vi "RelayBoard_ReadDi.vi"(9 "VISA资源名称":refnum<visa-resource-name>, 10 "比较值":bool, 11 "索引":i32) -> (2 "结果":bool, 3 "数组":bool[](array[boolean]))   [LabVIEW 2013]
panel:
  out "读取缓冲区":string
  # "深圳市德蓝新能源有限公司"
  # "X1"
  # "X2"
  # "X3"
  # "X4"
  # "X5"
  # "X6"
  # "X7"
  # "X8"
  # "X9"
  # "X10"
  # "X11"
  # "X12"
  # "X13"
  # "X14"
  # "X15"
  # "X16"
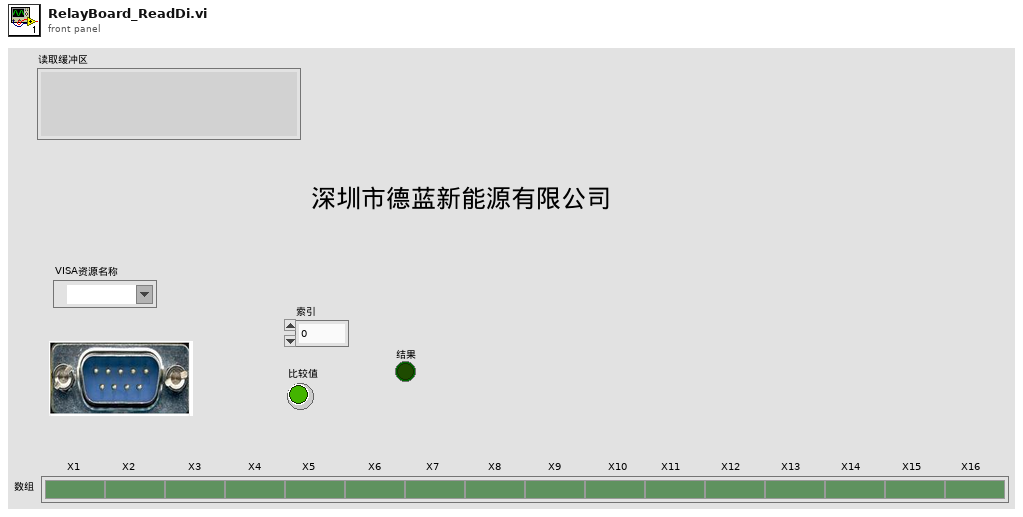
[diagram p1: front panel]
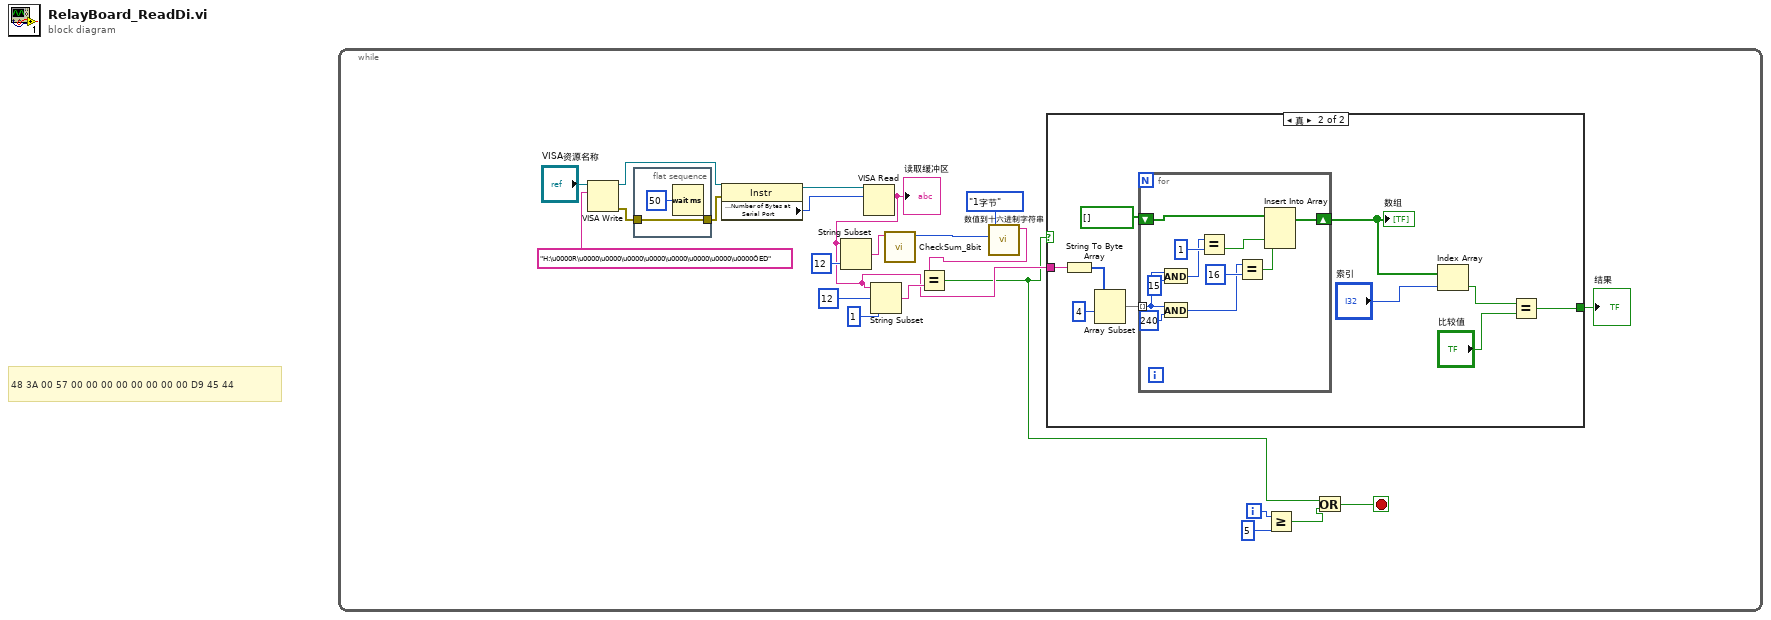
[diagram p0: block diagram]
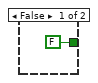
[diagram p2: hidden frame]
diagram:
  # "48 3A 00 57 00 00 00 00 00 00 00 00 D9 45 44"
  n1 = while {
    i -> [w5]
    stop <- w6 stop-if-true
    n2 = VISA Write(VISA resource name="VISA资源名称", write buffer="H:\u0000R\u0000\u0000\u0000\u0000\u0000\u0000\u0000\u0000ÔED" ("写入缓冲区")) -> (VISA resource name out=w7:refnum<visa-resource-name>, error out=w18:errorcluster)  [unwired: 1 in, 1 out]
    n3 = flat-sequence {
      tunnel: [w45] -> w19
      tunnel: w18 -> [w45]
      frame #0 {
        n4 = Wait (ms)(milliseconds to wait=u32 50 ("等待时间（毫秒）")) -> ()  [unwired: 1 out]
      }
    }
    n5 = property class="Instr"(reference=w7, error in=w19) -> (reference out=w22:refnum<visa-resource-name>, "Serial Settings:Number of Bytes at Serial Port"=w21:u32)  [unwired: 1 out]
    n6 = VISA Read(VISA resource name=w22, byte count=w21) -> (read buffer=w9:string)  [unwired: 1 in, 3 out]
    "读取缓冲区" <- w9
    n7 = String Subset(string=w9, length (rest)=12 ("长度（剩余）")) -> (substring=w13:string)  [unwired: 1 in]
    n8 = String Subset(string=w9, offset (0)=12 ("偏移量(0)"), length (rest)=1 ("长度（剩余）")) -> (substring=w14:string)
    n9 = call "CheckSum_8bit.vi"("字符串"=w13) -> ("和"=w11:u32)  [unwired: 10 in]
    n10 = call "数值到十六进制字符串.vi"("Numeric"=w11, "转换字节数"=enum16{"1字节", "2字节", "4字节", "3字节"}."1字节") -> ("转换结果"=w10:string)  [unwired: 8 in, 1 out]
    n11 = Equal?(x=w10, y=w14) -> (x = y?=w2:bool)
    n12 = case shown="真" w2 {
      tunnel: w9 -> [_ w33]
      tunnel: [FALSE w24] -> w1
      frame False {
      }
      frame True {
        n13 = String To Byte Array(string=w33) -> (unsigned byte array=w32:u8[])
        n14 = Array Subset(array=w32, index=4 ("索引")) -> (w30:u8[])  [unwired: 1 in]
        n15 = for {
          tunnel: w30 -> [w37] mode=indexing
          shift-right: [w39] -> w28
          shift-left: bool[] [] -> [w42]
          n16 = And(x=w37, y=u8 15) -> (x .and. y?=w35:u8)
          n17 = And(x=w37, y=u8 240) -> (x .and. y?=w34:u8)
          n18 = Equal?(x=w35, y=u8 1) -> (x = y?=w41:bool)
          n19 = Equal?(x=w34, y=u8 16) -> (x = y?=w40:bool)
          n20 = Insert Into Array(array=w42, new element #1=w41, new element #2=w40) -> (w39:bool[])  [unwired: 1 in]
        }
        "数组" <- w28
        n21 = Index Array(array=w28, index="索引") -> (element=w26:bool)
        n22 = Equal?(x=w26, y="比较值") -> (x = y?=w24:bool)
      }
    }
    "结果" <- w1
    n23 = Greater Or Equal?(x=w5, y=5) -> (x >= y?=w3:bool)
    n24 = Or(x=w2, y=w3) -> (x .or. y?=w6:bool)
  }
